vi "Handle Command.vi"(8 "error in (no error)":errorcluster, 9 "params in":variant, 10 "command":string, 11 "Inst.Transport in":refnum<class "Inst.Transport.lvclass">) -> (0 "error out":errorcluster, 1 "processed data":variant, 2 "command out":string, 3 "Inst.Transport out":refnum<class "Inst.Transport.lvclass">)   [LabVIEW 2019, in "Inst.Transport.lvclass"]
uses:
  Inst.Transport.lvclass
  Transport/Typedefs/Lockin_Sweep JSON--Cluster.ctl
  <userlib>/LevyLab/Lockin-Multichannel/Instrument.DAQ/Typedefs/Sweep.Channel--Cluster--Array.ctl
  <userlib>/LevyLab/Lockin-Multichannel/Instrument.DAQ/Typedefs/Sweep.Channel--Cluster.ctl
  <userlib>/LevyLab/Lockin-Multichannel/Instrument.DAQ/Typedefs/Sweep.Pattern--Enum.ctl
  Inst.Transport.lvclass/Inst.Transport.ctl
  Typedefs/ExptComments--RequestResponse--Cluster.ctl
  Typedefs/ExptFolder--RequestResponse--Cluster.ctl
  Transport/Transport.lvclass/Transport.ctl
  Typedefs/getStatus--Reply--Cluster.ctl
  Typedefs/Inst.Transport.Status--Enum.ctl
  b87ecf62-06e0-4335-967d-db4af97245ef.vi
  ab9961cd-e8f2-49a2-9a17-fbfd95da086c.vi
  583c3b72-57f9-4912-b162-c0263c95ab0a.vi
  b87ecf62-06e0-4335-967d-db4af97245ef.vi/835dc683-a2d1-4ce1-a25e-fe71450c48cd.vi
  b87ecf62-06e0-4335-967d-db4af97245ef.vi/1ab47e7e-2ffd-43be-8c69-6e3619e4b03c.vi
  ab9961cd-e8f2-49a2-9a17-fbfd95da086c.vi/cc82a950-28a9-4838-bc8d-5ba8078292ab.vi
  ab9961cd-e8f2-49a2-9a17-fbfd95da086c.vi/3297b0f4-d5ed-4960-b61d-4715e084f997.vi
  583c3b72-57f9-4912-b162-c0263c95ab0a.vi/5801969c-372f-4fc1-b827-4e2704f76ca0.vi
  583c3b72-57f9-4912-b162-c0263c95ab0a.vi/79e367b9-a887-4650-83ce-6b894da744c5.vi
  <vilib>/Utility/Data Type/Get Type Information.vi
  <vilib>/JDP Science/JSONtext/JSON text to Variant.vi
  <vilib>/JDP Science/JSONtext/LVClass Serializer/JSONtext LVClass Serializer.lvclass
  <userlib>/LevyLab/Instrument Framework/Instrument Types/SCPI/Instrument.SCPI.lvclass
  Typedefs/Inst.Transport.PublicCommands--Enum.ctl
  Typedefs/Inst.Transport.ProtectedCommands--Enum.ctl
  552737b8-b1ca-46ed-8e29-167e2822ff5d.vi
  25d97d38-0eab-472e-b12a-584ad5c8b013.vi
  <userlib>/LevyLab/Lockin-Multichannel/Instrument.DAQ/Instrument.DAQ.lvclass
  Transport/Transport.lvclass
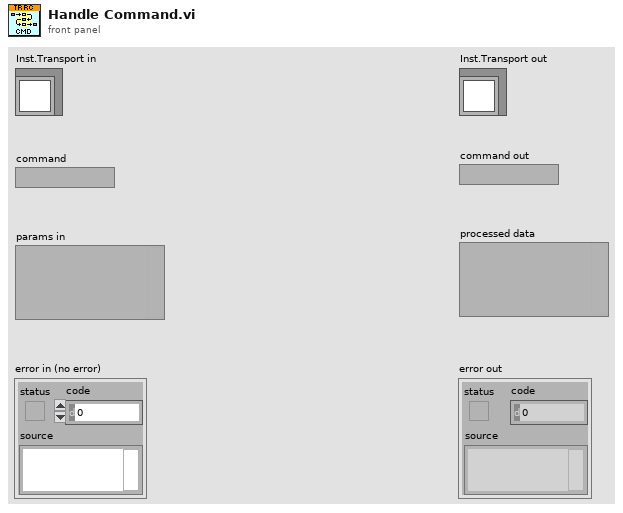
[diagram p1: front panel]
types:
  T1 = typedef "Transport.lvclass/Lockin_Sweep JSON--Cluster.ctl" = cluster{"initialWaitTime":dbl, "sweepTime":dbl, "Return to Start":bool, "sweepChannels":T2, "sweepTables":cluster{"Ch":i32, "Table":dbl[]}[]}
  T2 = typedef "Instrument.Lockin.lvlib/Instrument.DAQ.lvclass/Sweep.Channel--Cluster--Array.ctl" = T3[]
  T3 = typedef "Instrument.Lockin.lvlib/Instrument.DAQ.lvclass/Sweep.Channel--Cluster.ctl" = cluster{"Enable?":bool, "Channel":u16, "Start":dbl, "End":dbl, "Pattern":T4, "Table":dbl[]}
  T4 = typedef "Instrument.Lockin.lvlib/Instrument.DAQ.lvclass/Sweep.Pattern--Enum.ctl" = enum16{"Ramp /", "Ramp /\\", "Smooth Ramp _/", "Smooth Ramp _/\\_", "Table"}
  T5 = typedef "Inst.Transport.lvclass/ExptComments--RequestResponse--Cluster.ctl" = cluster{"comments":string}
  T6 = typedef "Inst.Transport.lvclass/ExptFolder--RequestResponse--Cluster.ctl" = cluster{"folder":string}
  T7 = typedef "Inst.Transport.lvclass/getStatus--Reply--Cluster.ctl" = cluster{"Status":T8}
  T8 = typedef "Inst.Transport.lvclass/Inst.Transport.Status--Enum.ctl" = enum16{"idle", "running"}
  T9 = typedef "Inst.Transport.lvclass/Inst.Transport.PublicCommands--Enum.ctl" = enum16{"startTransport", "stopTransport", "getStatus", "setExptFolder", "getExptFolder", "setExptComments", "getExptComments", "setExptParam", "appendExptParam", "clearExptParam", "setSweepConfig", "getSweepConfig", "setRefreshTime"}
  T10 = typedef "Inst.Transport.lvclass/Inst.Transport.ProtectedCommands--Enum.ctl" = enum16{"setStatus", "showUI", "hideUI"}
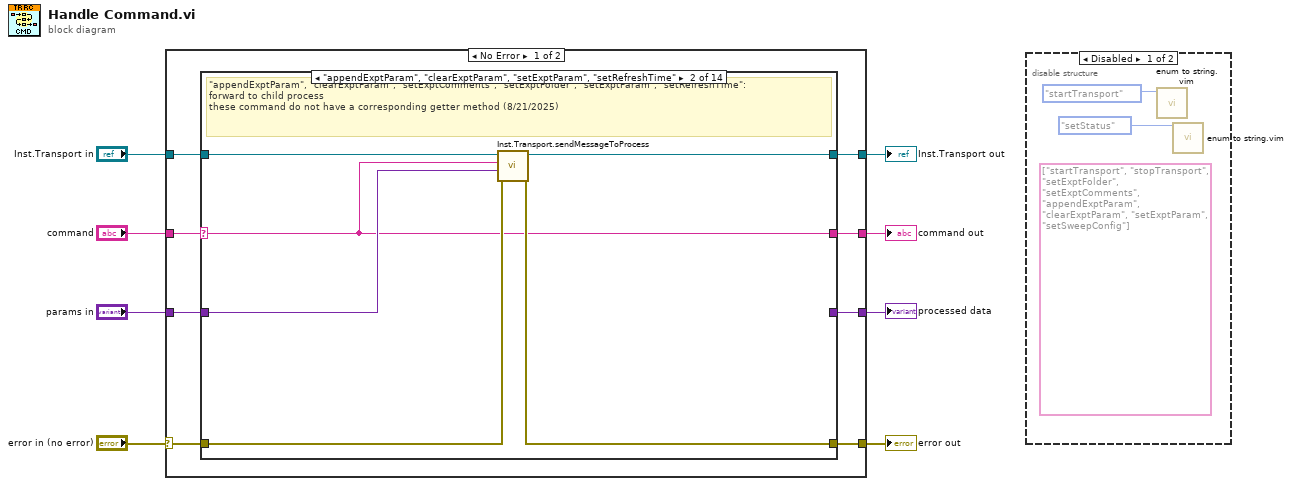
[diagram p0: block diagram]
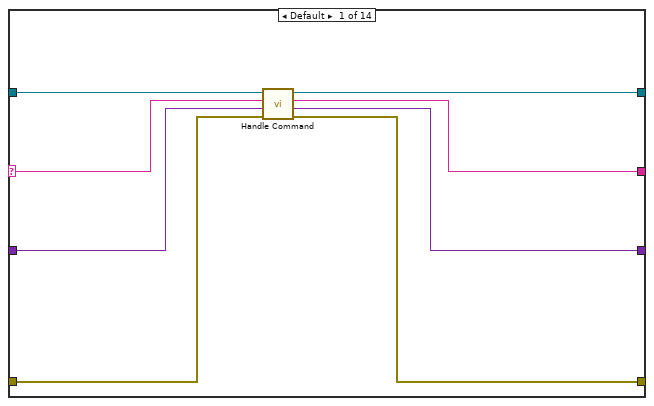
[diagram p3: hidden frame]
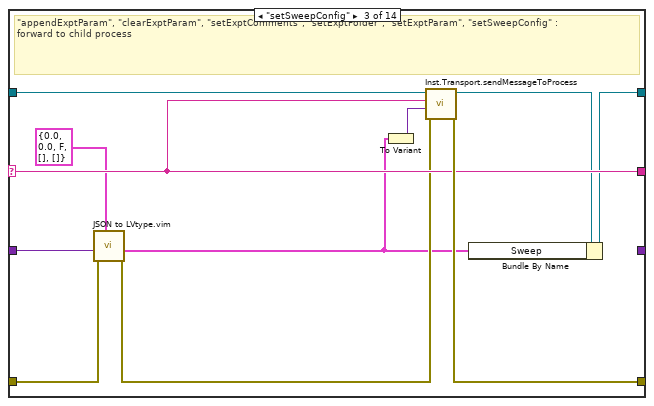
[diagram p4: hidden frame]
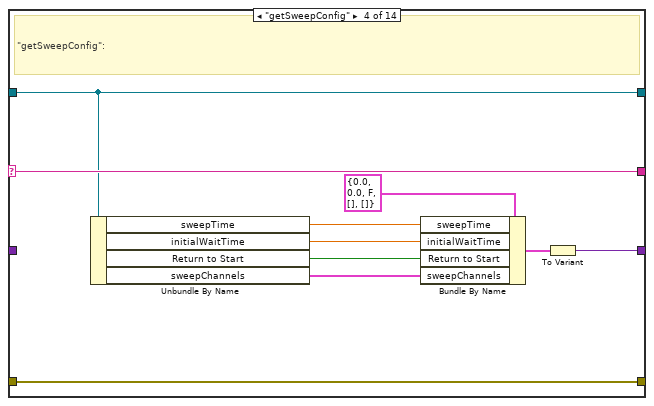
[diagram p5: hidden frame]
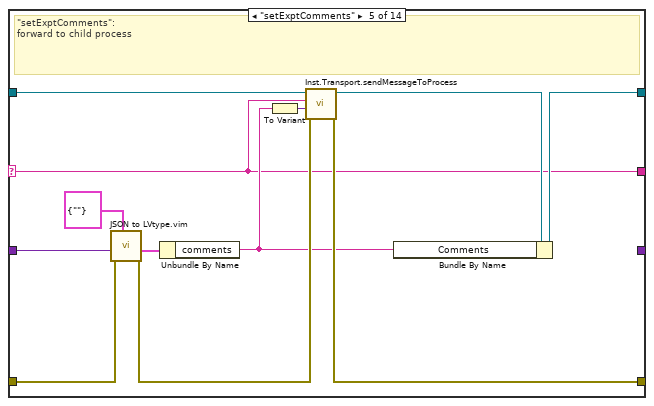
[diagram p6: hidden frame]
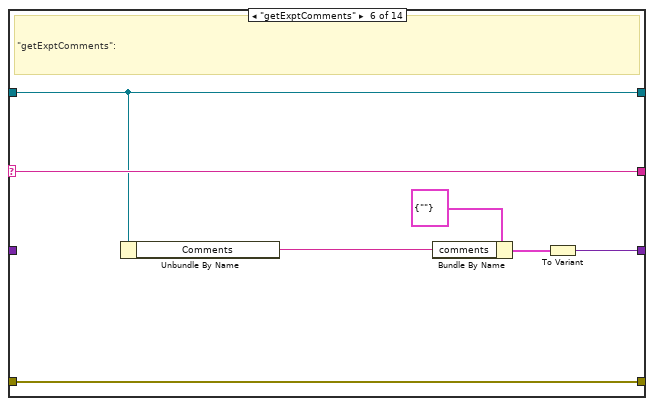
[diagram p7: hidden frame]
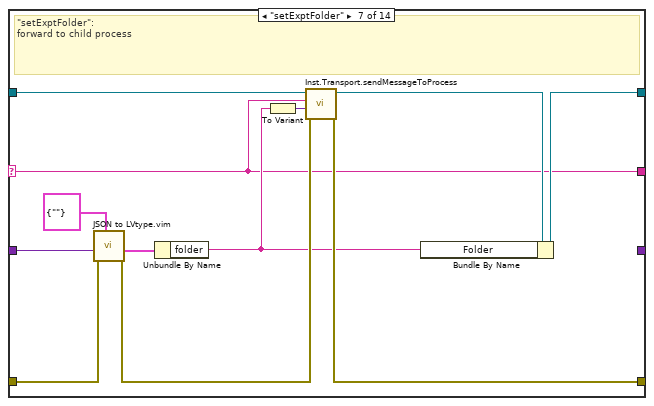
[diagram p8: hidden frame]
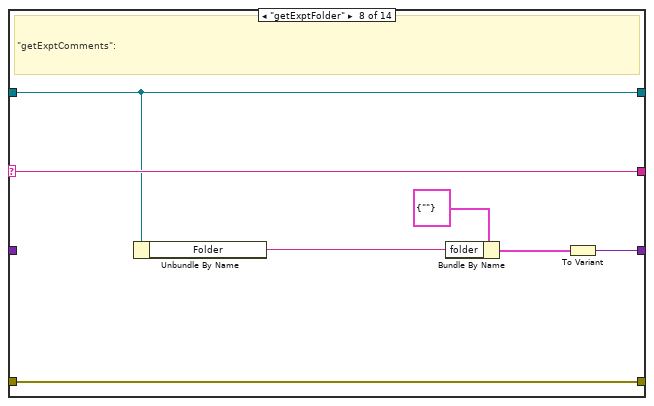
[diagram p9: hidden frame]
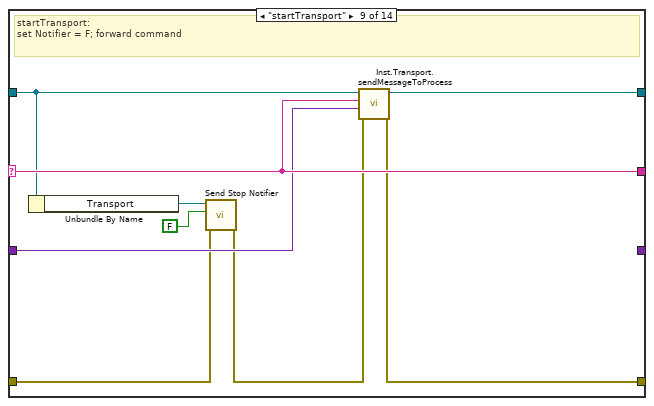
[diagram p10: hidden frame]
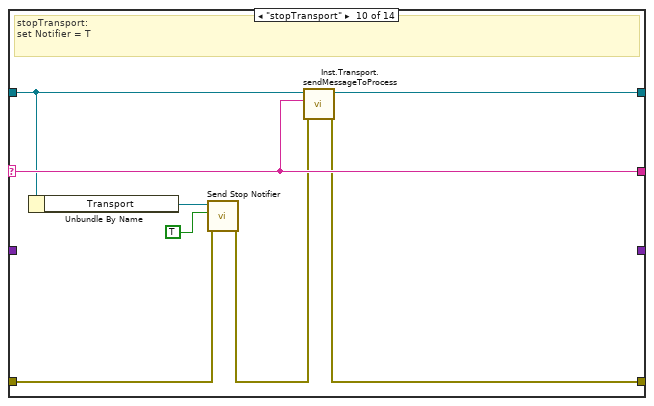
[diagram p11: hidden frame]
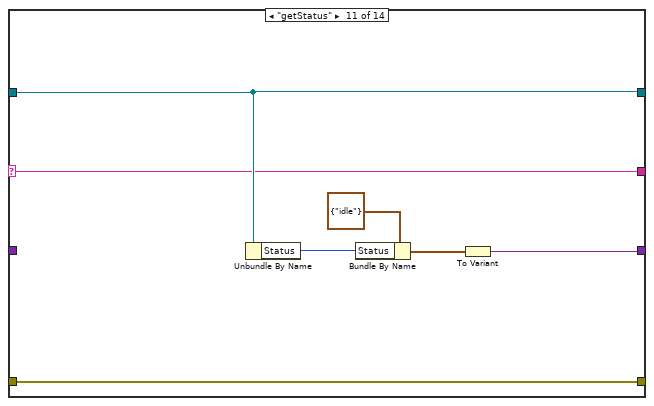
[diagram p12: hidden frame]
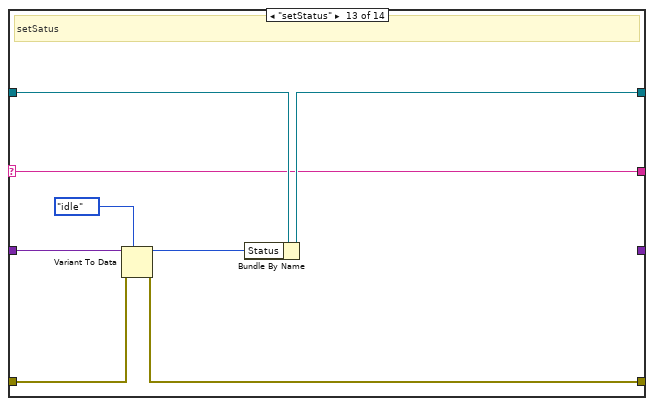
[diagram p14: hidden frame]
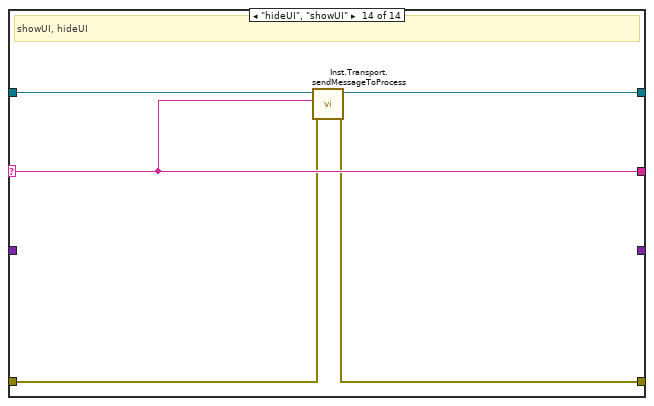
[diagram p15: hidden frame]
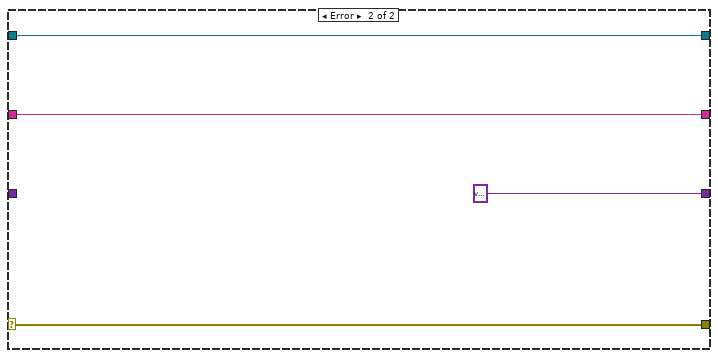
[diagram p16: hidden frame]
diagram:
  n1 = case shown="No Error" "error in (no error)" {
    selector: "error in (no error)" -> [w11 w132]
    tunnel: [w9 w132] -> w6
    tunnel: [w14 w131] -> w5
    tunnel: "Inst.Transport in" -> [w15 w131]
    tunnel: "command" -> [w16 w130]
    tunnel: [w13 variant ("Variant")] -> w3
    tunnel: "params in" -> [w10 _]
    tunnel: [w12 w130] -> w1
    frame No Error {
      n2 = case shown="\"appendExptParam\", \"clearExptParam\", \"setExptParam\", \"setRefreshTime\"" w16 {
        selector: w16 -> [w18 w26 w40 w51 w52 w70 w71 w89 w98 w105 w107 _ w116 w126]
        tunnel: w15 -> [w22 w30 w36 w48 w63 w66 w82 w86 w94 w104 w113 w115 w123 w128]
        tunnel: [w19 w25 w34 w48 w60 w66 w74 w86 w95 w106 w113 w115 w122 w127] -> w14
        tunnel: [w21 _ _ w46 _ w64 _ w83 _ _ w112 _ _ _] -> w13
        tunnel: w11 -> [w23 w29 w37 w47 w55 w65 w77 w85 w91 w101 w111 w114 w118 w125]
        tunnel: w10 -> [w24 w27 w39 _ w57 _ w76 _ w97 _ _ _ w120 _]
        tunnel: [w17 w26 w40 w51 w52 w70 w71 w89 w98 w105 w107 _ w116 w126] -> w12
        tunnel: [w20 w28 w41 w47 w62 w65 w81 w85 w96 w103 w111 w114 w117 w124] -> w9
        frame Default {
          n3 = call-parent "Handle Command.vi"("error in (no error)"=w23, "params in"=w24, "command"=w18, "Instrument in"=w22) -> ("error out"=w20:errorcluster, "processed data"=w21:variant, "command out"=w17:string, "Instrument out"=w19:refnum<class "Inst.Transport.lvclass">)  [unwired: 4 in]
        }
        frame "appendExptParam", "clearExptParam", "setExptParam", "setRefreshTime" {
          # "\"appendExptParam\", \"clearExptParam\", \"setExptComments\", \"setExptFolder\", \"setExptParam\", \"setRefreshTime\":\nforward to child process\nthese command do not have a corresponding getter method (8/21/2025)"
          n4 = call "Inst.Transport.sendMessageToProcess.vi"("error in (no error)"=w29, "Data"=w27, "Command"=w26, "Inst.Transport in"=w30) -> ("error out"=w28:errorcluster, "Inst.Transport out"=w25:refnum<class "Inst.Transport.lvclass">)  [unwired: 6 in]
        }
        frame "setSweepConfig" {
          # "\"appendExptParam\", \"clearExptParam\", \"setExptComments\", \"setExptFolder\", \"setExptParam\", \"setSweepConfig\" :\nforward to child process"
          n5 = call "JSON to LVtype.vim"("type"=T1 {"initialWaitTime"=0.0, "sweepTime"=0.0, "Return to Start"=FALSE, "sweepChannels"=[], "sweepTables"=[]} ("Lockin_sweep"), "error in (no error)"=w37, "JSON Data in"=w39) -> ("error out"=w38:errorcluster, "Data out"=w31:T1)  [unwired: 7 in]
          n6 = To Variant(anything=w31) -> (Variant=w33:variant)
          n7 = call "Inst.Transport.sendMessageToProcess.vi"("error in (no error)"=w38, "Data"=w33, "Command"=w40, "Inst.Transport in"=w36) -> ("error out"=w41:errorcluster, "Inst.Transport out"=w35:refnum<class "Inst.Transport.lvclass">)  [unwired: 6 in]
          n8 = Bundle By Name(cluster=w35, "Sweep"=w31) -> (w34:refnum<class "Inst.Transport.lvclass">)
        }
        frame "getSweepConfig" {
          # "\"getSweepConfig\":"
          n9 = Unbundle By Name(w48) -> ("sweepTime"=w50:dbl, "initialWaitTime"=w43:dbl, "Return to Start"=w44:bool, "sweepChannels"=w45:T2)
          n10 = Bundle By Name(cluster=T1 {"initialWaitTime"=0.0, "sweepTime"=0.0, "Return to Start"=FALSE, "sweepChannels"=[], "sweepTables"=[]} ("Lockin_sweep"), "sweepTime"=w50, "initialWaitTime"=w43, "Return to Start"=w44, "sweepChannels"=w45) -> (w49:T1)
          n11 = To Variant(anything=w49) -> (Variant=w46:variant)
        }
        frame "setExptComments" {
          # "\"setExptComments\":\nforward to child process"
          n12 = call "JSON to LVtype.vim"("type"=T5 {"comments"=""} ("setExptComments"), "error in (no error)"=w55, "JSON Data in"=w57) -> ("error out"=w56:errorcluster, "Data out"=w58:T5)  [unwired: 7 in]
          n13 = Unbundle By Name(w58) -> ("comments"=w54:string)
          n14 = To Variant(anything=w54) -> (Variant=w53:variant)
          n15 = call "Inst.Transport.sendMessageToProcess.vi"("error in (no error)"=w56, "Data"=w53, "Command"=w52, "Inst.Transport in"=w63) -> ("error out"=w62:errorcluster, "Inst.Transport out"=w61:refnum<class "Inst.Transport.lvclass">)  [unwired: 6 in]
          n16 = Bundle By Name(cluster=w61, "Comments"=w54) -> (w60:refnum<class "Inst.Transport.lvclass">)
        }
        frame "getExptComments" {
          # "\"getExptComments\":"
          n17 = Unbundle By Name(w66) -> ("Comments"=w68:string)
          n18 = Bundle By Name(cluster=T5 {"comments"=""} ("setExptComments"), "comments"=w68) -> (w67:T5)
          n19 = To Variant(anything=w67) -> (Variant=w64:variant)
        }
        frame "setExptFolder" {
          # "\"setExptFolder\":\nforward to child process"
          n20 = call "JSON to LVtype.vim"("type"=T6 {"folder"=""} ("setExptFolder"), "error in (no error)"=w77, "JSON Data in"=w76) -> ("error out"=w78:errorcluster, "Data out"=w79:T6)  [unwired: 7 in]
          n21 = Unbundle By Name(w79) -> ("folder"=w73:string)
          n22 = To Variant(anything=w73) -> (Variant=w72:variant)
          n23 = call "Inst.Transport.sendMessageToProcess.vi"("error in (no error)"=w78, "Data"=w72, "Command"=w71, "Inst.Transport in"=w82) -> ("error out"=w81:errorcluster, "Inst.Transport out"=w75:refnum<class "Inst.Transport.lvclass">)  [unwired: 6 in]
          n24 = Bundle By Name(cluster=w75, "Folder"=w73) -> (w74:refnum<class "Inst.Transport.lvclass">)
        }
        frame "getExptFolder" {
          # "\"getExptComments\":"
          n25 = Unbundle By Name(w86) -> ("Folder"=w88:string)
          n26 = Bundle By Name(cluster=T6 {"folder"=""} ("setExptFolder"), "folder"=w88) -> (w87:T6)
          n27 = To Variant(anything=w87) -> (Variant=w83:variant)
        }
        frame "startTransport" {
          # "startTransport:\nset Notifier = F; forward command"
          n28 = Unbundle By Name(w94) -> ("Transport"=w93:refnum<class "Transport.lvclass">)
          n29 = call "Send Stop Notifier.vi"("error in (no error)"=w91, "Stop [T]"=FALSE ("notification"), "Transport in"=w93) -> ("error out"=w90:errorcluster)  [unwired: 7 in, 1 out]
          n30 = call "Inst.Transport.sendMessageToProcess.vi"("error in (no error)"=w90, "Data"=w97, "Command"=w98, "Inst.Transport in"=w94) -> ("error out"=w96:errorcluster, "Inst.Transport out"=w95:refnum<class "Inst.Transport.lvclass">)  [unwired: 6 in]
        }
        frame "stopTransport" {
          # "stopTransport:\nset Notifier = T"
          n31 = Unbundle By Name(w104) -> ("Transport"=w102:refnum<class "Transport.lvclass">)
          n32 = call "Send Stop Notifier.vi"("error in (no error)"=w101, "Stop [T]"=TRUE ("notification"), "Transport in"=w102) -> ("error out"=w100:errorcluster)  [unwired: 7 in, 1 out]
          n33 = call "Inst.Transport.sendMessageToProcess.vi"("error in (no error)"=w100, "Command"=w105, "Inst.Transport in"=w104) -> ("error out"=w103:errorcluster, "Inst.Transport out"=w106:refnum<class "Inst.Transport.lvclass">)  [unwired: 7 in]
        }
        frame "getStatus" {
          n34 = Unbundle By Name(w113) -> ("Status"=w109:T8)
          n35 = Bundle By Name(cluster=T7 {"Status"=enum."idle"} ("getStatus"), "Status"=w109) -> (w108:T7)
          n36 = To Variant(anything=w108) -> (Variant=w112:variant)
        }
        frame "---Protected Methods---" {
        }
        frame "setStatus" {
          # "setSatus"
          n37 = Variant To Data(error in=w118, type=Inst.Transport.Status--Enum."idle" ("Status"), Variant=w120) -> (data=w121:T8, error out=w117:errorcluster)
          n38 = Bundle By Name(cluster=w123, "Status"=w121) -> (w122:refnum<class "Inst.Transport.lvclass">)
        }
        frame "hideUI", "showUI" {
          # "showUI, hideUI"
          n39 = call "Inst.Transport.sendMessageToProcess.vi"("error in (no error)"=w125, "Command"=w126, "Inst.Transport in"=w128) -> ("error out"=w124:errorcluster, "Inst.Transport out"=w127:refnum<class "Inst.Transport.lvclass">)  [unwired: 7 in]
        }
      }
    }
    frame Error {
    }
  }
  "error out" <- w6
  "Inst.Transport out" <- w5
  "command out" <- w1
  "processed data" <- w3
  n40 = disable-structure shown="Disabled" {
    frame Disabled {
      (unwired) string[] ["startTransport", "stopTransport", "setExptFolder", "setExptComments", "appendExptParam", "clearExptParam", "setExptParam", "setSweepConfig"] ("Commands")
      n41 = call "enum to string.vim"("enum in"=Inst.Transport.PublicCommands--Enum."startTransport" ("PublicCommands")) -> ()  [unwired: 9 in, 2 out]
      n42 = call "enum to string.vim"("enum in"=Inst.Transport.ProtectedCommands--Enum."setStatus" ("ProtectedCommands")) -> ()  [unwired: 9 in, 2 out]
    }
    frame Enabled {
    }
  }
